vi "Update Scores.vi"(10 "Winning Vote":string, 11 "map in":map{i32, T2}(c390)) -> (2 "Score Table":T1[](array[typedef]), 3 "map out":map{i32, T2}(c390))   [LabVIEW 2019]
doc: "Updates the voters score tally."
uses:
  SubVIs/Voter Info.ctl
  Scoreboard Entry.ctl
  <vilib>/Utility/miscctls.llb/LVMapReplaceAction.ctl
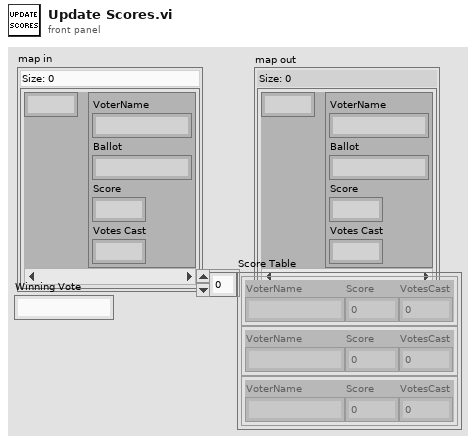
[diagram p1: front panel]
types:
  T1 = typedef "Scoreboard Entry.ctl" = cluster{"VoterName":string, "Score":i32, "VotesCast":i32}
  T2 = typedef "Voter Info.ctl" = cluster{"VoterName":string, "Ballot":string, "Score":i32, "Votes Cast":i32}
  T3 = typedef "LVMapReplaceAction.ctl" = enum32{"Modify Entry only if found", "Add or Modify Entry", "Delete Entry"}
  T4 = cluster{"Score":i32, cluster{"VoterID":i32, "VoterInfo":T2}}
  T5 = cluster{"Score":i32, cluster{"VoterID":i32, "VoterInfo":T2}}[]
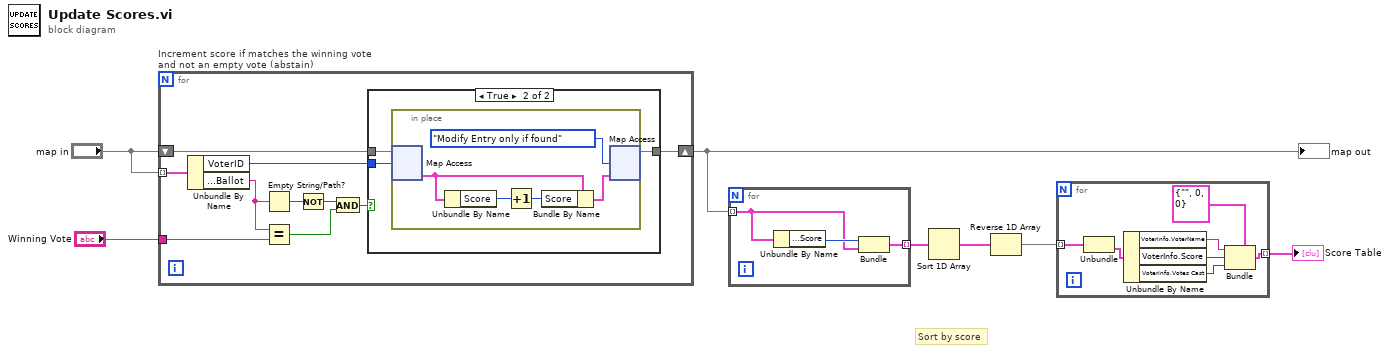
[diagram p0: block diagram]
diagram:
  # "Sort by score"
  n1 = for "Increment score if matches the winning vote and not an empty vote (abstain)" {
    shift-right: [w10] -> w5
    shift-left: "map in" -> [w17]
    tunnel: "map in" -> [w16] mode=indexing
    tunnel: "Winning Vote" -> [w14]
    n2 = Unbundle By Name(w16) -> ("VoterID"=w15:i32, "VoterInfo.Ballot"=w13:string)
    n3 = Empty String/Path?(string/path=w13) -> (empty?=w12:bool)
    n4 = Equal?(x=w13, y=w14) -> (x = y?=w11:bool)
    n5 = Not(x=w12) -> (.not. x?=w8:bool)
    n6 = And(x=w8, y=w11) -> (x .and. y?=w9:bool)
    n7 = case shown="True" w9 {
      tunnel: w17 -> [w18 w21]
      tunnel: w15 -> [_ w20]
      tunnel: [w18 w19] -> w10
      frame False {
      }
      frame True {
        n8 = in-place {
          n9 = in-place-map #1(w21, w20) -> (w25:T2)  [unwired: 1 in, 1 out]
          n10 = Unbundle By Name(w25) -> ("Score"=w26:i32)
          n11 = Increment(x=w26) -> (x+1=w24:i32)
          n12 = Bundle By Name(cluster=w25, "Score"=w24) -> (w23:T2)
          n13 = in-place-map #1(w23, LVMapReplaceAction."Modify Entry only if found" ("action")) -> (w19:map{i32, T2})  [unwired: 2 out]
        }
      }
    }
  }
  "map out" <- w5
  n14 = for {
    tunnel: w5 -> [w28] mode=indexing
    tunnel: [w27] -> w4 mode=indexing
    n15 = Unbundle By Name(w28) -> ("VoterInfo.Score"=w29:i32)
    n16 = Bundle("Score"=w29, w28) -> (w27:T4)  [unwired: 1 in]
  }
  n17 = Sort 1D Array(array=w4) -> (sorted array=w3:T5)
  n18 = Reverse 1D Array(array=w3) -> (reversed array=w1:T5)
  n19 = for {
    tunnel: w1 -> [w36] mode=indexing
    tunnel: [w32] -> w2 mode=indexing
    n20 = Unbundle(w36) -> (w35:cluster{"VoterID":i32, "VoterInfo":T2})  [unwired: 1 out]
    n21 = Unbundle By Name(w35) -> ("VoterInfo.VoterName"=w34:string, "VoterInfo.Score"=w33:i32, "VoterInfo.Votes Cast"=w30:i32)
    n22 = Bundle(cluster=T1 {"VoterName"="", "Score"=0, "VotesCast"=0} ("Score"), "VoterName"=w34, "Score"=w33, "VotesCast"=w30) -> (w32:T1)
  }
  "Score Table" <- w2
